vi "SetOperationMode.vi"(0 "VISA resource name in":refnum<visa-resource-name>, 5 "ON/OFF":bool, 6 "Operation Mode Status":T1, 11 "error in":errorcluster, 12 "Laser":bool, 13 "Power":bool, 14 "Guide laser":bool=TRUE) -> (4 "VISA resource name out":refnum<visa-resource-name>, 10 "Message":string, 15 "error out":errorcluster)   [LabVIEW 2014]
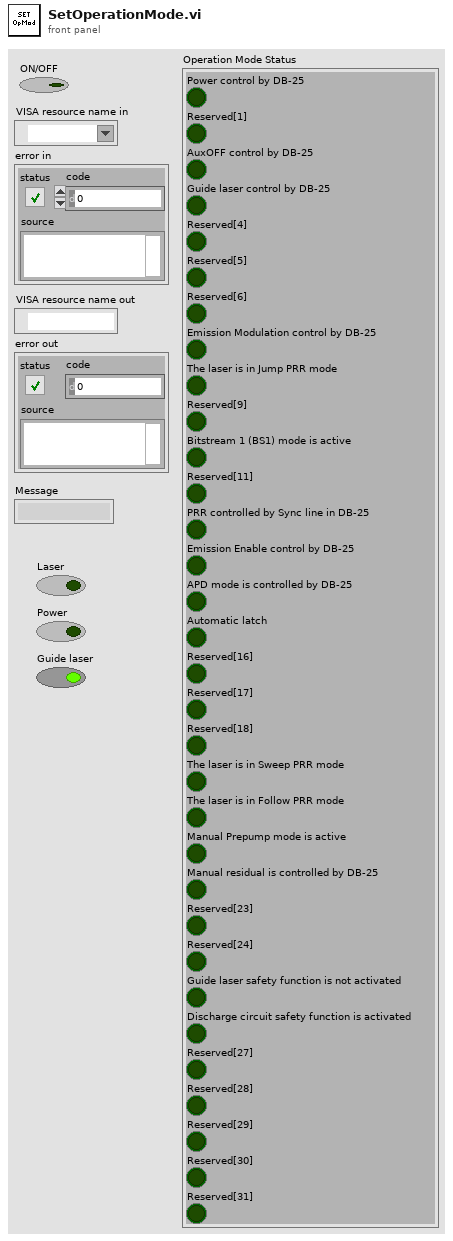
[diagram p1: front panel]
types:
  T1 = cluster{"Power control by DB-25":bool, "Reserved[1]":bool, "AuxOFF control by DB-25":bool, "Guide laser control by DB-25":bool, "Reserved[4]":bool, "Reserved[5]":bool, "Reserved[6]":bool, "Emission Modulation control by DB-25":bool, "The laser is in Jump PRR mode":bool, "Reserved[9]":bool, "Bitstream 1 (BS1) mode is active":bool, "Reserved[11]":bool, "PRR controlled by Sync line in DB-25":bool, "Emission Enable control by DB-25":bool, "APD mode is controlled by DB-25":bool, "Automatic latch":bool, "Reserved[16]":bool, "Reserved[17]":bool, "Reserved[18]":bool, "The laser is in Sweep PRR mode":bool, "The laser is in Follow PRR mode":bool, "Manual Prepump mode is active":bool, "Manual residual is controlled by DB-25":bool, "Reserved[23]":bool, "Reserved[24]":bool, "Guide laser safety function is not activated":bool, "Discharge circuit safety function is activated":bool, "Reserved[27]":bool, "Reserved[28]":bool, "Reserved[29]":bool, "Reserved[30]":bool, "Reserved[31]":bool}
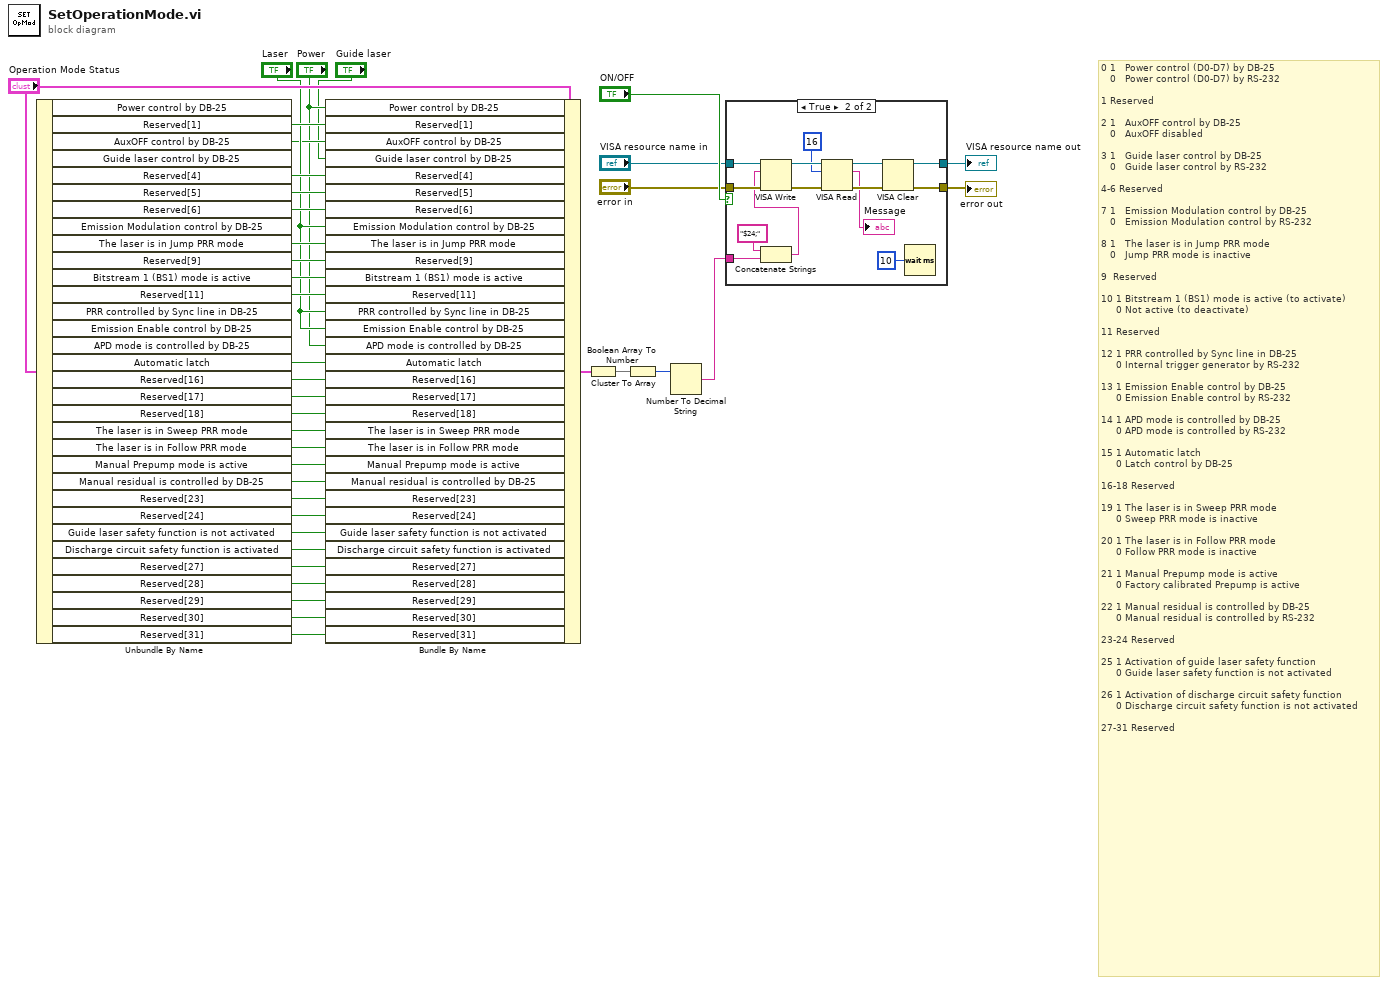
[diagram p0: block diagram]
diagram:
  # "0 1   Power control (D0-D7) by DB-25\n   0   Power control (D0-D7) by RS-232\n\n1 Reserved\n\n2 1   AuxOFF control by DB-25\n   0   AuxOFF disabled\n\n3 1   Guide laser control by DB-25\n   0   Guide laser control by RS-232\n\n4-6 Reserved\n\n7 1   Emission Modulation control by DB-25\n   0   Emission Modulation control by RS-232\n\n8 1   The laser is in Jump PRR mode\n   0   Jump PRR mode is inactive\n\n9  Reserved\n\n10 1 Bitstream 1 (BS1) mode is active (to activate)\n     0 Not active (to deactivate)\n\n11 Reserved\n\n12 1 PRR controlled by Sync line in DB-25\n     0 Internal trigger generator by RS-232\n\n13 1 Emission Enable control by DB-25\n     0 Emission Enable control by RS-232\n\n14 1 APD mode is controlled by DB-25\n     0 APD mode is controlled by RS-232\n\n15 1 Automatic latch\n     0 Latch control by DB-25\n\n16-18 Reserved\n\n19 1 The laser is in Sweep PRR mode\n     0 Sweep PRR mode is inactive\n\n20 1 The laser is in Follow PRR mode\n     0 Follow PRR mode is inactive\n\n21 1 Manual Prepump mode is active\n     0 Factory calibrated Prepump is active\n\n22 1 Manual residual is controlled by DB-25\n     0 Manual residual is controlled by RS-232\n\n23-24 Reserved\n\n25 1 Activation of guide laser safety function\n     0 Guide laser safety function is not activated\n\n26 1 Activation of discharge circuit safety function\n     0 Discharge circuit safety function is not activated\n\n27-31 Reserved"
  n1 = Unbundle By Name("Operation Mode Status") -> ("Reserved[1]"=w34:bool, "AuxOFF control by DB-25"=w4:bool, "Reserved[4]"=w33:bool, "Reserved[5]"=w32:bool, "Reserved[6]"=w31:bool, "The laser is in Jump PRR mode"=w15:bool, "Reserved[9]"=w30:bool, "Bitstream 1 (BS1) mode is active"=w14:bool, "Reserved[11]"=w29:bool, "Automatic latch"=w13:bool, "Reserved[16]"=w28:bool, "Reserved[17]"=w27:bool, "Reserved[18]"=w26:bool, "The laser is in Sweep PRR mode"=w12:bool, "The laser is in Follow PRR mode"=w11:bool, "Manual Prepump mode is active"=w10:bool, "Manual residual is controlled by DB-25"=w3:bool, "Reserved[23]"=w24:bool, "Reserved[24]"=w23:bool, "Guide laser safety function is not activated"=w8:bool, "Discharge circuit safety function is activated"=w7:bool, "Reserved[27]"=w22:bool, "Reserved[28]"=w21:bool, "Reserved[29]"=w20:bool, "Reserved[30]"=w19:bool, "Reserved[31]"=w18:bool)  [unwired: 6 out]
  n2 = Bundle By Name(cluster="Operation Mode Status", "Power control by DB-25"="Power", "Reserved[1]"=w34, "AuxOFF control by DB-25"=w4, "Guide laser control by DB-25"="Guide laser", "Reserved[4]"=w33, "Reserved[5]"=w32, "Reserved[6]"=w31, "Emission Modulation control by DB-25"="Laser", "The laser is in Jump PRR mode"=w15, "Reserved[9]"=w30, "Bitstream 1 (BS1) mode is active"=w14, "Reserved[11]"=w29, "PRR controlled by Sync line in DB-25"="Laser", "Emission Enable control by DB-25"="Laser", "APD mode is controlled by DB-25"="Power", "Automatic latch"=w13, "Reserved[16]"=w28, "Reserved[17]"=w27, "Reserved[18]"=w26, "The laser is in Sweep PRR mode"=w12, "The laser is in Follow PRR mode"=w11, "Manual Prepump mode is active"=w10, "Manual residual is controlled by DB-25"=w3, "Reserved[23]"=w24, "Reserved[24]"=w23, "Guide laser safety function is not activated"=w8, "Discharge circuit safety function is activated"=w7, "Reserved[27]"=w22, "Reserved[28]"=w21, "Reserved[29]"=w20, "Reserved[30]"=w19, "Reserved[31]"=w18) -> (w17:T1)
  n3 = Cluster To Array(cluster=w17) -> (array=w16:bool[])
  n4 = Boolean Array To Number(Boolean array=w16) -> (number=w6:u32)
  n5 = Number To Decimal String(number=w6) -> (decimal integer string=w5:string)  [unwired: 1 in]
  n6 = case shown="True" "ON/OFF" {
    tunnel: "VISA resource name in" -> [w41 w53]
    tunnel: "error in" -> [w40 w52]
    tunnel: [w41 w49] -> w36
    tunnel: [w40 w48] -> w35
    tunnel: w5 -> [_ w43]
    frame False {
    }
    frame True {
      n7 = Concatenate Strings("$24;" ("write buffer"), w43) -> (w42:string)
      n8 = VISA Write(VISA resource name=w53, write buffer=w42, error in (no error)=w52) -> (VISA resource name out=w54:refnum<visa-resource-name>, error out=w55:errorcluster)  [unwired: 1 out]
      n9 = VISA Read(VISA resource name=w54, byte count=u32 16, error in (no error)=w55) -> (VISA resource name out=w51:refnum<visa-resource-name>, read buffer=→"Message":string, error out=w50:errorcluster)  [unwired: 1 out]
      n10 = VISA Clear(VISA resource name=w51, error in (no error)=w50) -> (VISA resource name out=w49:refnum<visa-resource-name>, error out=w48:errorcluster)
      n11 = Wait (ms)(milliseconds to wait=u32 10) -> ()  [unwired: 1 out]
    }
  }
  "VISA resource name out" <- w36
  "error out" <- w35
